vi "Special_Processing.vi"(6 "cluster in":T1, 8 "error in (no error)":errorcluster, 9 "Terminal Map In":map{string, T3}(c390), 10 "Wires":T2[](array[typedef]), 11 "MultiDiagramStructure in":refnum<class "MultiDiagramStructure.lvclass">) -> (0 "error out":errorcluster, 1 "Terminal Map Out":map{string, T3}(c390), 2 "Wires out":T2[](array[typedef]), 3 "MultiDiagramStructure out":refnum<class "MultiDiagramStructure.lvclass">)   [LabVIEW 2025, in "MultiDiagramStructure.lvclass"]
uses:
  MultiDiagramStructure.lvclass
  wire.ctl
  Terminal.ctl
  bd.ctl
  Node/Node.lvclass
  MultiDiagramStructure.lvclass/MultiDiagramStructure.ctl
  <vilib>/regexp/Match Regular Expression.xnode
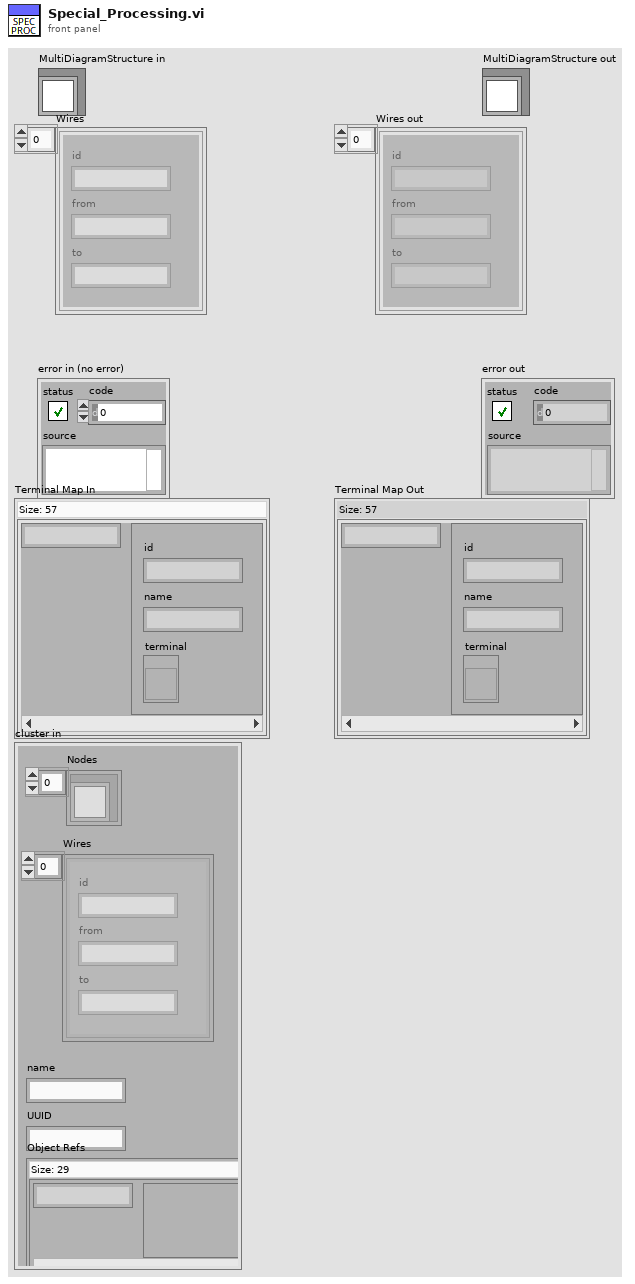
[diagram p1: front panel]
types:
  T1 = typedef "bd.ctl" = cluster{"Nodes":refnum<class "Node.lvclass">[], "Wires":T2[], "name":string, "UUID":string, "Object Refs":map{string, variant}}
  T2 = typedef "wire.ctl" = cluster{"id":string, "from":string, "to":string}
  T3 = typedef "Terminal.ctl" = cluster{"id":string, "name":string, "terminal":refnum<vi>}
  T4 = typedef "Tunnel.ctl" = cluster{"OuterUUID":T3, "InnerUUIDs":T3[]}
  T5 = typedef "Subdiagram.ctl" = cluster{"diagram":refnum<vi>, "selector":string, "uuid":string}
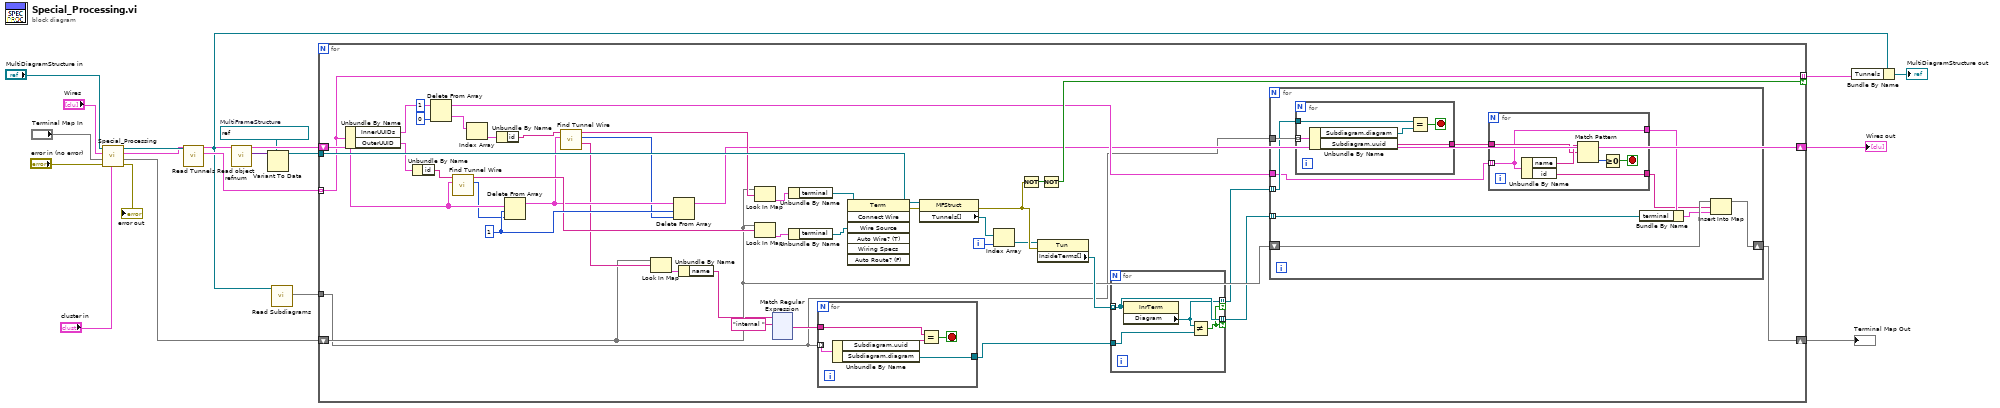
[diagram p0: block diagram]
diagram:
  w7 = refnum<vi> refnum  # MultiFrameStructure
  n1 = call-parent "Special_Processing.vi"("cluster in"="cluster in", "error in (no error)"="error in (no error)", "Terminal Map In"="Terminal Map In", "Wires"="Wires", "Node in"="MultiDiagramStructure in") -> ("error out"=→"error out":errorcluster, "Terminal Map Out"=w14:map{string, T3}, "Wires out"=w15:T2[], "Node out"=w16:refnum<class "MultiDiagramStructure.lvclass">)  [unwired: 3 in]
  n2 = call-dynamic "Read Tunnels.vi"("MultiDiagramStructure in"=w16) -> ("Tunnels"=w4:T4[], "MultiDiagramStructure out"=w2:refnum<class "MultiDiagramStructure.lvclass">)  [unwired: 8 in, 1 out]
  n3 = call-dynamic "Read object refnum.vi"("Node in"=w2) -> ("object refnum"=w8:variant)  [unwired: 8 in, 2 out]
  n4 = Variant To Data(type=w7, Variant=w8) -> (data=w6:refnum<vi>)  [unwired: 1 in, 1 out]
  n5 = call-dynamic "Read Subdiagrams.vi"("MultiDiagramStructure in"=w2) -> ("Subdiagrams"=w1:map{u64, T5})  [unwired: 8 in, 2 out]
  n6 = for {
    shift-right: [w54] -> w11
    shift-left: w14 -> [w33]
    tunnel: w4 -> [w46] mode=indexing
    tunnel: w6 -> [w57]
    shift-right: [w26] -> w12
    shift-left: w15 -> [w52]
    tunnel: [w46] -> w3 mode=indexing if=w43
    tunnel: w1 -> [w21]
    i -> [w56]
    w53 = 1 ("length")
    n7 = Unbundle By Name(w46) -> ("InnerUUIDs"=w55:T3[], "OuterUUID"=w25:T3)
    n8 = Unbundle By Name(w25) -> ("id"=w24:string)
    n9 = Delete From Array(array=w55, length=1, index=0) -> (deleted portion=w36:T3[], array with subset deleted=w39:T3[])
    n10 = call "Find Tunnel Wire.vi"("Wires"=w52, "termUUID"=w24) -> ("Index"=w51:i32, "destination terminal"=w50:string)  [unwired: 7 in, 1 out]
    n11 = Index Array(array=w36) -> (element=w23:T3)  [unwired: 1 in]
    n12 = Unbundle By Name(w23) -> ("id"=w22:string)
    n13 = Delete From Array(array=w52, length=w53, index=w51) -> (array with subset deleted=w49:T2[])  [unwired: 1 out]
    n14 = call "Find Tunnel Wire.vi"("Wires"=w49, "termUUID"=w22) -> ("other_end"=w34:string, "Index"=w48:i32, "destination terminal"=w47:string)  [unwired: 7 in]
    n15 = Look In Map(map=w33, key=w34) -> (value=w32:T3)  [unwired: 1 in, 1 out]
    n16 = Delete From Array(array=w49, length=w53, index=w48) -> (array with subset deleted=w26:T2[])  [unwired: 1 out]
    n17 = Unbundle By Name(w32) -> ("name"=w31:string)
    n18 = Look In Map(map=w33, key=w47) -> (value=w60:T3)  [unwired: 1 in, 1 out]
    n19 = Look In Map(map=w33, key=w50) -> (value=w61:T3)  [unwired: 1 in, 1 out]
    n20 = xnode "Match Regular Expression"("input string"=w31, "regular expression"="internal ") -> ("after match"=w29:string)  [unwired: 4 in, 4 out]
    n21 = Unbundle By Name(w60) -> ("terminal"=w59:refnum<vi>)
    n22 = Unbundle By Name(w61) -> ("terminal"=w40:refnum<vi>)
    n23 = for {
      tunnel: w21 -> [w66] mode=indexing
      tunnel: w29 -> [w64]
      tunnel: [w62] -> w28
      stop <- w63 stop-if-true
      n24 = Unbundle By Name(w66) -> ("Subdiagram.uuid"=w65:string, "Subdiagram.diagram"=w62:refnum<vi>)
      n25 = Equal?(x=w64, y=w65) -> (x = y?=w63:bool)
    }
    n26 = invoke class="Term" method="Connect Wire"(reference=w59, "Wire Source"=w40) -> (error out=w58:errorcluster)  [unwired: 5 in, 6 out]
    n27 = property class="MFStruct"(reference=w57, error in=w58) -> (error out=w45:errorcluster, "Tunnels[]"=w41:refnum<vi>[])  [unwired: 1 out]
    n28 = Index Array(array=w41, index=w56) -> (element=w42:refnum<vi>)
    n29 = Not(x=w45) -> (.not. x?=w44:bool)
    n30 = property class="Tun"(reference=w42, error in=w45) -> ("InsideTerms[]"=w35:refnum<vi>[])  [unwired: 2 out]
    n31 = Not(x=w44) -> (.not. x?=w43:bool)
    n32 = for {
      tunnel: w35 -> [w186] mode=indexing
      tunnel: [w186] -> w27 mode=indexing if=w184
      tunnel: w28 -> [w187]
      tunnel: [w185] -> w20 mode=indexing if=w184
      n33 = property class="InrTerm"(reference=w186) -> ("Diagram"=w185:refnum<vi>)  [unwired: 1 in, 2 out]
      n34 = Not Equal?(x=w185, y=w187) -> (x != y?=w184:bool)
    }
    n35 = for {
      tunnel: w39 -> [w191]
      tunnel: w27 -> [w197] mode=indexing
      shift-right: [w196] -> w54
      shift-left: w33 -> [w195]
      tunnel: w21 -> [w194]
      tunnel: w20 -> [w193] mode=indexing
      n36 = for {
        tunnel: w194 -> [w208] mode=indexing
        tunnel: w193 -> [w205]
        tunnel: [w204] -> w192
        stop <- w207 stop-if-true
        n37 = Unbundle By Name(w208) -> ("Subdiagram.diagram"=w206:refnum<vi>, "Subdiagram.uuid"=w204:string)
        n38 = Equal?(x=w205, y=w206) -> (x = y?=w207:bool)
      }
      n39 = for {
        tunnel: w192 -> [w202]
        tunnel: w191 -> [w199] mode=indexing
        tunnel: [w199] -> w190
        tunnel: [w198] -> w188
        stop <- w200 stop-if-true
        n40 = Unbundle By Name(w199) -> ("name"=w203:string, "id"=w198:string)
        n41 = Match Pattern(string=w203, regular expression=w202) -> (offset past match=w201:i32)  [unwired: 1 in, 3 out]
        n42 = Greater Or Equal To 0?(x=w201) -> (x >= 0?=w200:bool)
      }
      n43 = Bundle By Name(cluster=w190, "terminal"=w197) -> (w189:T3)
      n44 = Insert Into Map(map in=w195, key=w188, value=w189) -> (map out=w196:map{string, T3})  [unwired: 2 out]
    }
  }
  "Wires out" <- w12
  "Terminal Map Out" <- w11
  n45 = Bundle By Name(cluster=w2, "Tunnels"=w3) -> (→"MultiDiagramStructure out":refnum<class "MultiDiagramStructure.lvclass">)
